vi "HIOKI PW3390 Conf Averaging.vi"(0 "VISA Resource":refnum<visa-resource-name>, 1 "Set/Query (F: Set)":bool, 5 "Averaging (0: OFF)":T1(ring), 11 "error in (no error)":errorcluster, 12 "OPC query (T: ON)":bool=TRUE, 13 "Error Out (F: Off)":bool) -> (4 "VISA Resource out":refnum<visa-resource-name>, 6 "Averaging out":T1(ring), 15 "error out":errorcluster)   [LabVIEW 2009]
doc: "Set/Query\n Set: Send the setting commands for the device.\n Query: Query the setting of the device.\n\nAveraging\n Sets the averaging setting. The averaging process will start again when the average setting is changed."
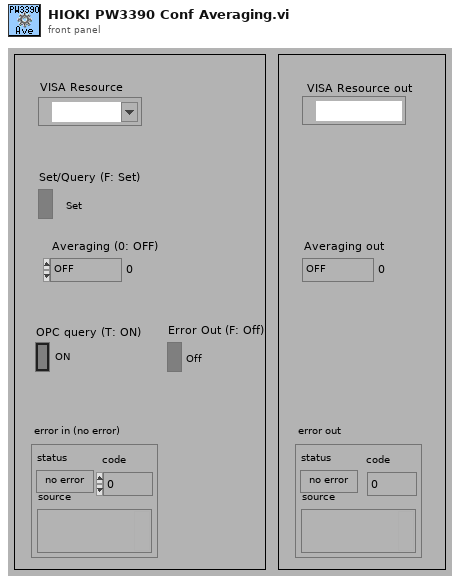
[diagram p1: front panel]
types:
  T1 = enum16{"OFF", "FAST", "MID", "SLOW", "SLOW2", "SLOW3"}
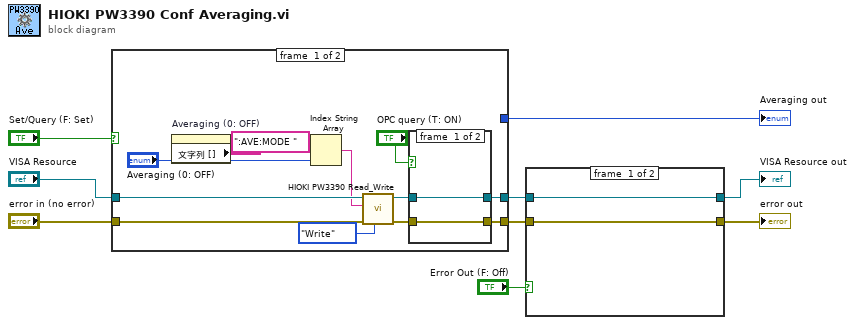
[diagram p0: block diagram]
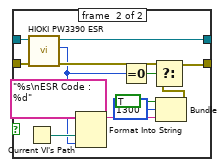
[diagram p2: hidden frame]
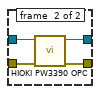
[diagram p3: hidden frame]
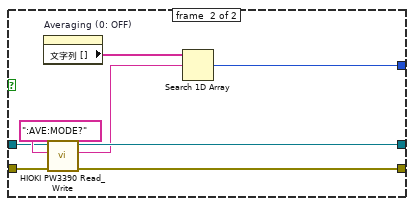
[diagram p4: hidden frame]
diagram:
  n1 = case shown="FALSE" "Set/Query (F: Set)" {
    tunnel: "error in (no error)" -> [w19 w31]
    tunnel: [w10 w34] -> w4
    tunnel: "VISA Resource" -> [w20 w32]
    tunnel: [w11 w33] -> w5
    tunnel: [_ w28] -> w7
    frame #0 {
      n2 = property on="Averaging (0: OFF)" class="Enum （指定）"() -> ("文字列 []"=w15:string[])  [unwired: 2 in, 2 out]
      n3 = Index String Array(1:"Averaging (0: OFF)", 2:w15, 3:":AVE:MODE ") -> (0:w16:string)
      n4 = call <instrlib>:"HIOKI PW3390 Read_Write.vi"("Read/Write"=enum16{"Read", "Write"}."Write", "error in (no error)"=w19, "data in"=w16, "VISA Resource"=w20) -> ("error out"=w13:errorcluster, "VISA Resource out"=w12:refnum<visa-resource-name>)  [unwired: 5 in, 1 out]
      n5 = case shown="TRUE" "OPC query (T: ON)" {
        tunnel: [w23 w27] -> w11
        tunnel: [w22 w26] -> w10
        tunnel: w13 -> [w22 w25]
        tunnel: w12 -> [w23 w24]
        frame #0 {
        }
        frame #1 {
          n6 = call <instrlib>:"HIOKI PW3390 OPC.vi"("error in (no error)"=w25, "VISA Resource"=w24) -> ("error out"=w26:errorcluster, "VISA Resource out"=w27:refnum<visa-resource-name>)  [unwired: 7 in, 1 out]
        }
      }
    }
    frame #1 {
      n7 = property on="Averaging (0: OFF)" class="Enum （指定）"() -> ("文字列 []"=w29:string[])  [unwired: 2 in, 2 out]
      n8 = call <instrlib>:"HIOKI PW3390 Read_Write.vi"("error in (no error)"=w31, "data in"=":AVE:MODE?", "VISA Resource"=w32) -> ("error out"=w34:errorcluster, "data out"=w30:string, "VISA Resource out"=w33:refnum<visa-resource-name>)  [unwired: 6 in]
      n9 = Search 1D Array(1D array=w29, element=w30) -> (index of element=w28:i32)  [unwired: 1 in]
    }
  }
  "Averaging out" <- w7
  n10 = case shown="TRUE" "Error Out (F: Off)" {
    tunnel: w5 -> [w37 w50]
    tunnel: w4 -> [w36 w49]
    tunnel: [w36 w39] -> w3
    tunnel: [w37 w48] -> w1
    frame #0 {
    }
    frame #1 {
      n11 = Current VI's Path() -> (path=w46:path)
      n12 = call <instrlib>:"HIOKI PW3390 ESR.vi"("error in (no error)"=w49, "VISA Resource"=w50) -> ("error out"=w40:errorcluster, "Output Value"=w38:u8, "VISA Resource out"=w48:refnum<visa-resource-name>)  [unwired: 6 in, 1 out]
      n13 = Format Into String(format string="%s\nESR Code : %d", w46, w38) -> (resulting string=w42:string)  [unwired: 2 in, 1 out]
      n14 = Equal To 0?(x=w38) -> (x = 0?=w47:bool)
      n15 = Bundle("status"=TRUE, "code"=1300, w42) -> (w41:cluster{"status":bool, "code":i32, string})  [unwired: 1 in]
      n16 = Select(t=w40, s=w47, f=w41) -> (s? t:f=w39:errorcluster)
    }
  }
  "error out" <- w3
  "VISA Resource out" <- w1
